vi "ArmGetMotorOutput.vi"() -> (1 "ExtendMotorOutput":dbl, 2 "LiftMotorOutput":dbl)   [LabVIEW 2020]
doc: "Get motor outputs for arm from global varibles\nOutputs:\n--RotateMoterOutput--double--degrees--\n--LiftMotorOutput--double--degrees--\n--ExtendMotorOutput--double--inches--"
uses:
  ArmGlobal.vi
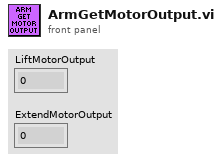
[diagram p1: front panel]
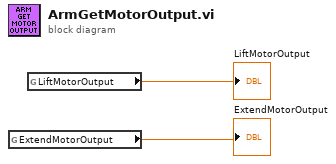
[diagram p0: block diagram]
diagram:
  n1 = global read "ArmGlobal.vi" "ExtendMotorOutput"() -> (→"ExtendMotorOutput":dbl)
  n2 = global read "ArmGlobal.vi" "LiftMotorOutput"() -> (→"LiftMotorOutput":dbl)
